vi "02READ REG-simple.vi"() -> (0 "error out":errorcluster, 1 "Pass":string, 2 "Nombre":string)   [LabVIEW 2010]
uses:
  <vilib>/registry/registry.llb/Registry RtKey.ctl
  <vilib>/registry/registry.llb/Read Registry Value Simple.vi
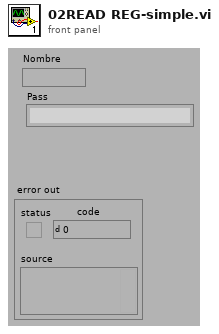
[diagram p1: front panel]
types:
  T1 = typedef "Registry RtKey.ctl" = enum32{"HKEY_CLASSES_ROOT", "HKEY_CURRENT_USER", "HKEY_LOCAL_MACHINE", "HKEY_USERS", "HKEY_PERFORMANCE_DATA", "HKEY_CURRENT_CONFIG", "HKEY_DYN_DATA"}
  T2 = typedef "Registry refnum.ctl" = refnum<k1>
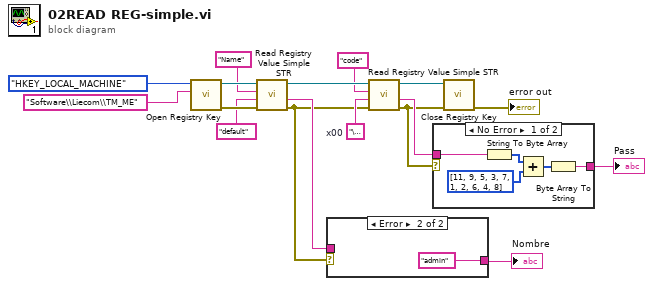
[diagram p0: block diagram]
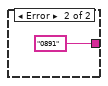
[diagram p3: hidden frame]
diagram:
  w10 = "\u0000"  # x00
  n1 = call <vilib>:"Open Registry Key.vi"("subkey"="Software\\Liecom\\TM_ME", "root key (HKEY_LOCAL_MACHINE)"=Registry_RtKey."HKEY_LOCAL_MACHINE") -> ("error out"=w15:errorcluster, "refnum out"=w14:T2)  [unwired: 8 in]
  n2 = call-poly <vilib>:"Read Registry Value Simple STR.vi"("error in (no error)"=w15, "default data"="default", "value"="Name", "refnum"=w14) -> ("error out"=w1:errorcluster, "String/Binary data"=w4:string, "refnum out"=w12:T2)  [unwired: 2 in, 1 out]
  n3 = case shown="Error" w1 {
    tunnel: w4 -> [w18 _]
    tunnel: [w18 "admin" ("string")] -> w3
    frame No Error {
    }
    frame Error {
    }
  }
  "Nombre" <- w3
  n4 = call-poly <vilib>:"Read Registry Value Simple STR.vi"("error in (no error)"=w1, "default data"=w10, "value"="code", "refnum"=w12) -> ("error out"=w2:errorcluster, "String/Binary data"=w8:string, "refnum out"=w6:T2)  [unwired: 2 in, 1 out]
  n5 = case shown="No Error" w2 {
    tunnel: w8 -> [w22 _]
    tunnel: [w20 "0891" ("string")] -> w5
    frame No Error {
      n6 = String To Byte Array(string=w22) -> (unsigned byte array=w24:u8[])
      n7 = Add(x=w24, y=u8[] [11, 9, 5, 3, 7, 1, 2, 6, 4, 8]) -> (x+y=w21:u8[])
      n8 = Byte Array To String(unsigned byte array=w21) -> (string=w20:string)
    }
    frame Error {
    }
  }
  "Pass" <- w5
  n9 = call <vilib>:"Close Registry Key.vi"("error in (no error)"=w2, "refnum"=w6) -> ("error out"=→"error out":errorcluster)  [unwired: 5 in]
